vi "ImageMagic Append Wrapper.vi"(8 "error in (no error)":errorcluster, 9 "Append Method":T1, 10 "Output File":path, 11 "Input Files":path[](array[path])) -> (0 "error out":errorcluster)   [LabVIEW 2020, in "VIDiffImageMagic.lvlib"]
uses:
  VIDiffImageMagic.lvlib
  Append Method.ctl
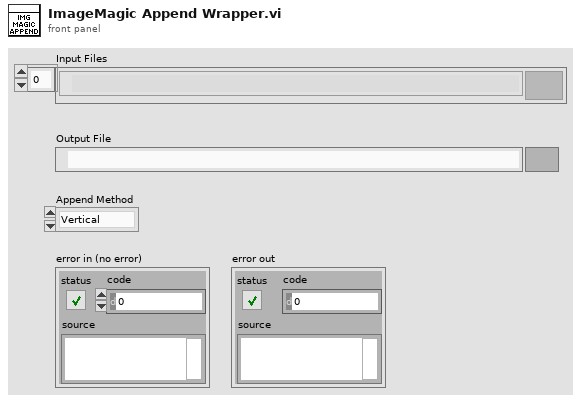
[diagram p1: front panel]
types:
  T1 = typedef "VIDiffImageMagic.lvlib/Append Method.ctl" = enum16{"Vertical", "Horizontal"}
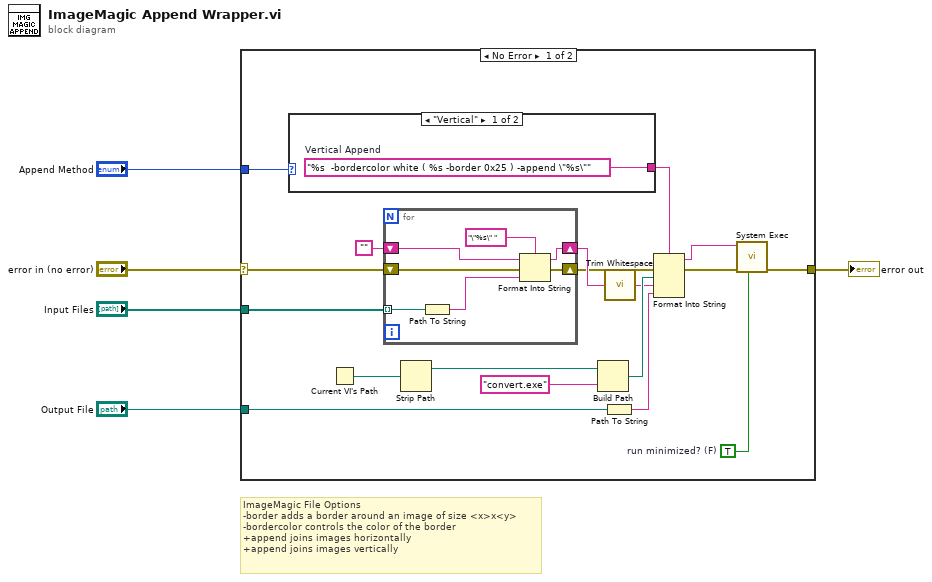
[diagram p0: block diagram]
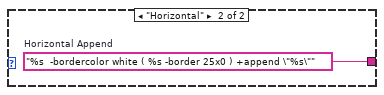
[diagram p2: hidden frame]
diagram:
  # "ImageMagic File Options\n-border adds a border around an image of size <x>x<y>\n-bordercolor controls the color of the border\n+append joins images horizontally\n+append joins images vertically"
  n1 = case shown="No Error" "error in (no error)" {
    selector: "error in (no error)" -> [w9 w33]
    tunnel: [w18 w33] -> w5
    tunnel: "Output File" -> [w15 _]
    tunnel: "Input Files" -> [w10 _]
    tunnel: "Append Method" -> [w8 _]
    frame No Error {
      w20 = TRUE  # run minimized? (F)
      n2 = case shown="\"Vertical\"" w8 {
        tunnel: [w24 w25] -> w13
        frame "Vertical" {
          w24 = "%s  -bordercolor white ( %s -border 0x25 ) -append \"%s\""  # Vertical Append
        }
        frame "Horizontal" {
          w25 = "%s  -bordercolor white ( %s -border 25x0 ) +append \"%s\""  # Horizontal Append
        }
      }
      n3 = Current VI's Path() -> (path=w7:path)
      n4 = for {
        tunnel: w10 -> [w32] mode=indexing
        shift-right: [w29] -> w14
        shift-left: "" -> [w28]
        shift-right: [w26] -> w12
        shift-left: w9 -> [w27]
        n5 = Path To String(path=w32) -> (string=w30:string)
        n6 = Format Into String(format string="\"%s\" ", initial string=w28, error in=w27, w30) -> (resulting string=w29:string, error out=w26:errorcluster)
      }
      n7 = Strip Path(path=w7) -> (stripped path=w6:path)  [unwired: 1 out]
      n8 = Build Path(base path=w6, name or relative path="convert.exe") -> (appended path=w23:path)
      n9 = Path To String(path=w15) -> (string=w16:string)
      n10 = call <vilib>:"Trim Whitespace.vi"("string"=w14) -> ("trimmed string"=w22:string)  [unwired: 1 in]
      n11 = Format Into String(format string=w13, error in=w12, w23, w22, w16) -> (resulting string=w19:string, error out=w17:errorcluster)  [unwired: 1 in]
      n12 = call <vilib>:"System Exec.vi"("run minimized? (F)"=w20, "error in (no error)"=w17, "command line"=w19) -> ("error out"=w18:errorcluster)  [unwired: 5 in, 3 out]
    }
    frame Error {
    }
  }
  "error out" <- w5
